vi "Set OP and Post OP Measurements.vi"(8 "error in (no error)":errorcluster, 11 "Input Power Measurement in":refnum<class "Input Power Measurement.lvclass">) -> (0 "error out":errorcluster, 3 "Input Power Measurement out":refnum<class "Input Power Measurement.lvclass">)   [LabVIEW 2018, in "Input Power Measurement.lvlib" / "Input Power Measurement.lvclass"]
uses:
  Input Power Measurement.lvclass
  Plugins/Measurements/Servo MSMT.lvlibp/Servo MSMT.lvclass
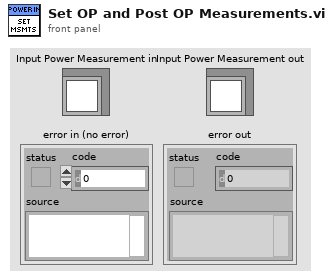
[diagram p1: front panel]
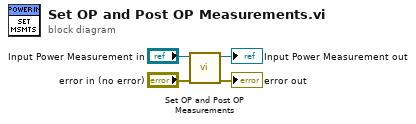
[diagram p0: block diagram]
diagram:
  n1 = call-parent "Set OP and Post OP Measurements.vi"("error in (no error)"="error in (no error)", "Servo MSMT in"="Input Power Measurement in") -> ("error out"=→"error out":errorcluster, "Servo MSMT out"=→"Input Power Measurement out":refnum<class "Input Power Measurement.lvclass">)  [unwired: 8 in]
